vi "ReadCoeffs.vi"(11 "CoeFile in":refnum<class "CoeFile.lvclass">) -> (1 "shift":i32, 2 "Coeffs":fxp<+/-,18,18>[](array[numeric]), 3 "CoeFile out":refnum<class "CoeFile.lvclass">)   [LabVIEW 2013, in "CoeFile.lvclass"]
uses:
  CoeFile.lvclass
  CoeFile.lvclass/CoeFile.ctl
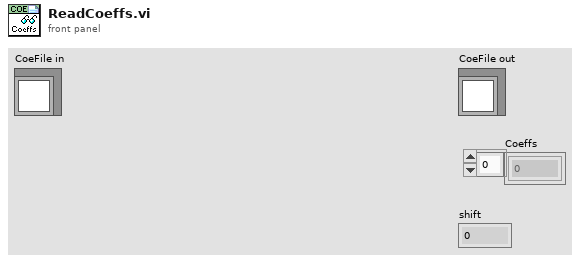
[diagram p1: front panel]
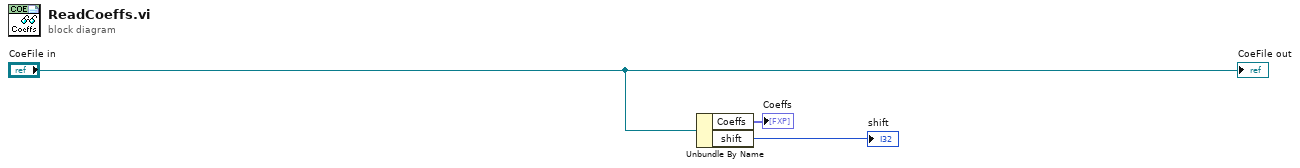
[diagram p0: block diagram]
diagram:
  n1 = Unbundle By Name("CoeFile in") -> ("Coeffs"=→"Coeffs":fxp<+/-,18,18>[], "shift"=→"shift":i32)
  "CoeFile out" <- "CoeFile in"
